vi "VCS Get Protocol Stack Name Selection.vi"(0 "device in":T1={"deviceName"="EPOS2", "protocolStackName"="", "interfaceName"="", "portName"=""}, 5 "startOfSelection":i32, 11 "error in (no error)":errorcluster) -> (4 "device out":T1={"deviceName"="EPOS2", "protocolStackName"="", "interfaceName"="", "portName"=""}, 6 "endOfSelection":i32, 8 "protocolStackNameSel":string, 15 "error out":errorcluster)   [LabVIEW 2010]
doc: "<B>VCS Get Protocol Stack Name Selection</B> returns all available protocol stack names."
uses:
  Resources/EposCmd.dll
  Resources/EposCmd64.dll
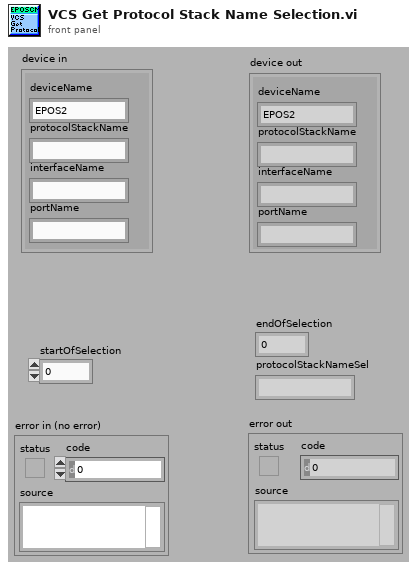
[diagram p1: front panel]
types:
  T1 = cluster{"deviceName":string, "protocolStackName":string, "interfaceName":string, "portName":string}
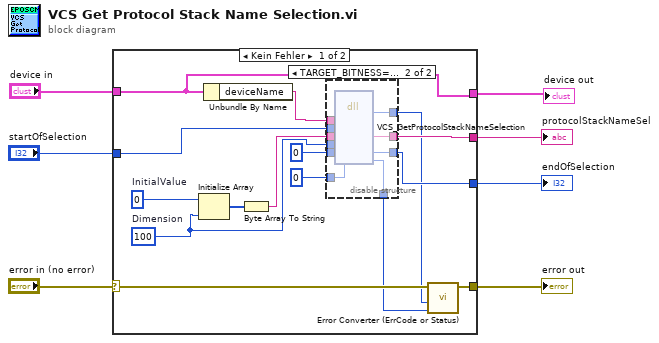
[diagram p0: block diagram]
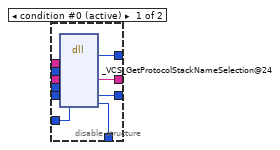
[diagram p2: hidden frame]
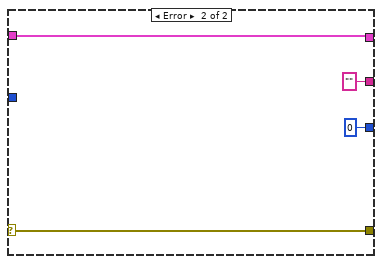
[diagram p3: hidden frame]
diagram:
  n1 = case shown="Kein Fehler" "error in (no error)" {
    selector: "error in (no error)" -> [w19 w46]
    tunnel: [w18 w46] -> w6
    tunnel: "startOfSelection" -> [w22 _]
    tunnel: [w21 "" ("pProtocolStackNameSel")] -> w4
    tunnel: [w20 0 ("pEndOfSelection")] -> w3
    tunnel: "device in" -> [w15 w44]
    tunnel: [w15 w44] -> w1
    frame No Error {
      w11 = u8 0  # InitialValue
      w9 = 100  # Dimension
      n2 = Initialize Array(w11, w9) -> (w12:u8[])
      n3 = Unbundle By Name(w15) -> ("deviceName"=w16:string)
      n4 = Byte Array To String(unsigned byte array=w12) -> (string=w10:string)
      n5 = disable-structure shown="TARGET_BITNESS==64" {
        disable-tunnel: w22 -> [w32 w42]
        disable-tunnel: [w31 w41] -> w21
        disable-tunnel: [w30 w40] -> w20
        disable-tunnel: [w29 w39] -> w17
        disable-tunnel: w16 -> [w28 w38]
        disable-tunnel: 0 ("pEndOfSelection") -> [w27 w37]
        disable-tunnel: u32 0 ("pErrorCode") -> [w26 w36]
        disable-tunnel: w10 -> [w25 w35]
        disable-tunnel: w9 -> [w24 w34]
        disable-tunnel: [w23 w33] -> w8
        frame condition #0 (active) {
          n6 = dll-call lib="C:/Sources/LabView/maxon EPOS/Resources/EposCmd.*" fn="_VCS_GetProtocolStackNameSelection@24"("DeviceName"=w28, "StartOfSelection"=w32, "pProtocolStackNameSel"=w25, "MaxStrSize"=w24, "pEndOfSelection"=w27, "pErrorCode"=w26) -> (w23:i32, "pProtocolStackNameSel"=w31:string, "pEndOfSelection"=w30:i32, "pErrorCode"=w29:u32)  [unwired: 6 in, 2 out]
        }
        frame condition #1 {
          n7 = dll-call lib="C:/setup/Resources/EposCmd64.*" fn="VCS_GetProtocolStackNameSelection" ("EposCmd.dll:_VCS_GetProtocolStackNameSelection@24")("DeviceName"=w38, "StartOfSelection"=w42, "pProtocolStackNameSel"=w35, "MaxStrSize"=w34, "pEndOfSelection"=w37, "pErrorCode"=w36) -> ("Rückgabetyp"=w33:i32, "pProtocolStackNameSel"=w41:string, "pEndOfSelection"=w40:i32, "pErrorCode"=w39:u32)  [unwired: 6 in, 2 out]
        }
      }
      n8 = call "Error Converter (ErrCode or Status).vi"("error code"=w17, "return type"=w8, "error in (no error)"=w19) -> ("error out"=w18:errorcluster)  [unwired: 7 in]
    }
    frame Error {
    }
  }
  "protocolStackNameSel" <- w4
  "endOfSelection" <- w3
  "error out" <- w6
  "device out" <- w1
